vi "New Stainless Correction Pop Up 2016.vi"(3 "New Feet\n of Stainless\n(Count)":i32, 5 "Depth to \nWater Table\nInput":dbl) -> (0 "Feet of\nStainless to be\nUsed (Count)":i32, 2 "Depth to \nWater Table\nOutput":dbl)   [LabVIEW 2016]
doc: "This vi allows the clinician to input the starting flexion. It used in order to derive a flexion correction."
uses:
  KPRO_lv2015/Kpro Globals.vi
panel:
  out "Original Feet\n of Stainless\n(Count)":i32
  in  "stop":bool
  in  "Increment Stainless":bool
  in  "Stainless OK As Is":bool
  in  "Correct Stainless":bool
  # "Please Choose \nto Correct, Increment, or to \nLeave Feet of Stainless as is"
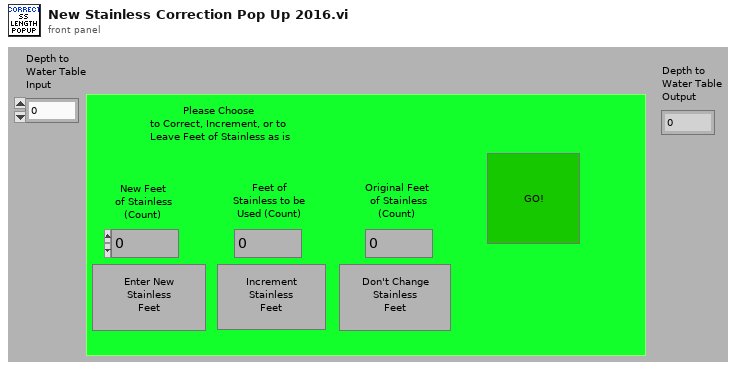
[diagram p1: front panel]
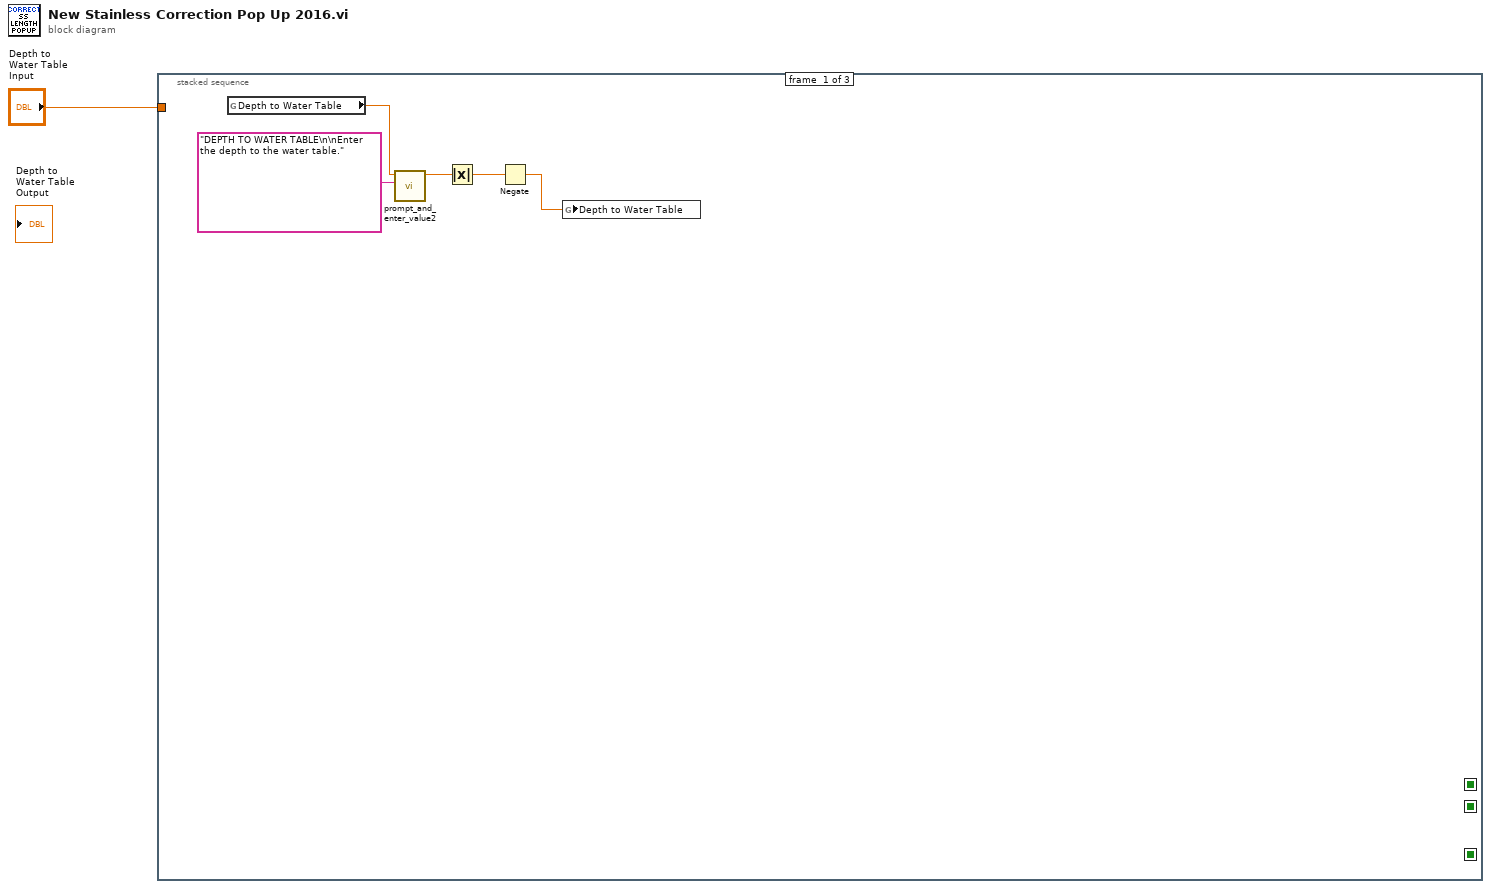
[diagram p0: block diagram]
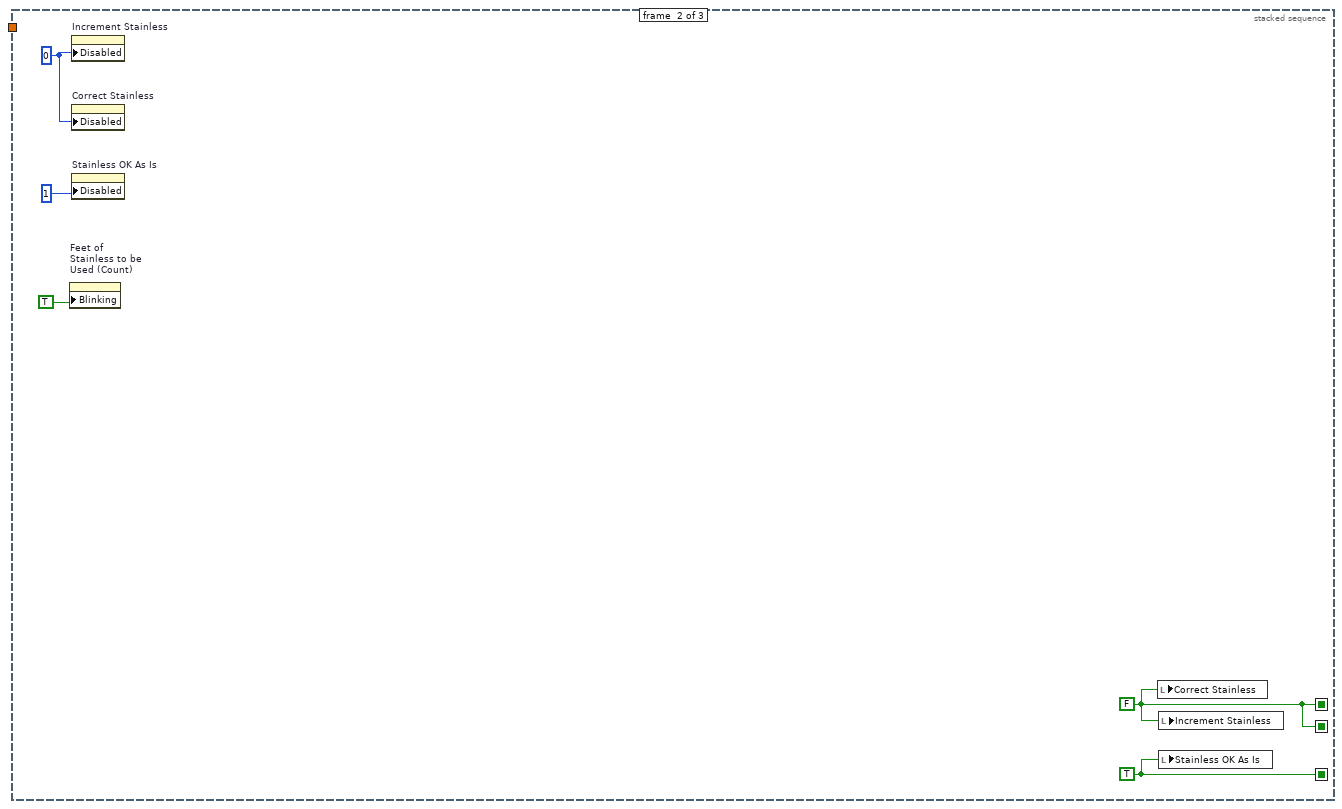
[diagram p2: hidden frame]
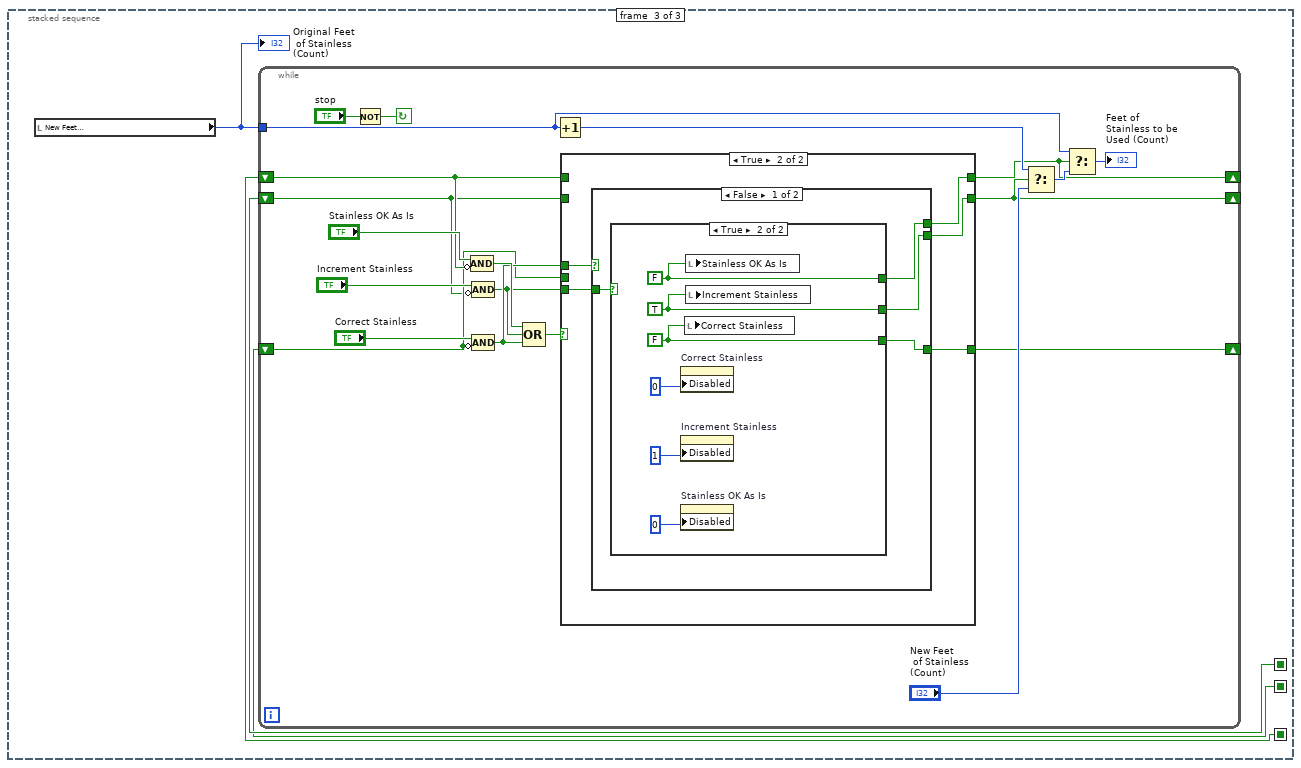
[diagram p3: hidden frame]
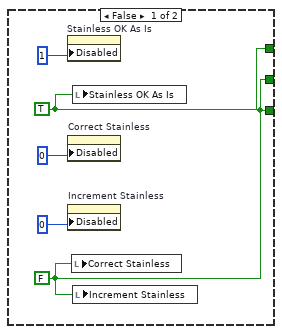
[diagram p5: hidden frame]
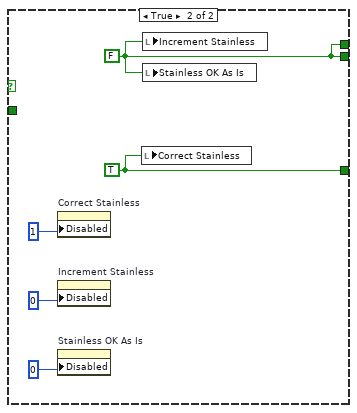
[diagram p6: hidden frame]
diagram:
  n1 = stacked-sequence {
    seq-local: [_ w10 _] -> [_ _ w13]
    seq-local: [_ w10 _] -> [_ _ w14]
    seq-local: [_ w11 _] -> [_ _ w15]
    tunnel: "Depth to \nWater Table\nInput" -> [_ _ _]
    frame #0 {
      n2 = global read "Kpro Globals.vi" "Depth to Water Table"() -> (w6:dbl)
      n3 = call "prompt_and_enter_value2.vi"("prompt_IN"="DEPTH TO WATER TABLE\n\nEnter the depth to the water table." ("prompt"), "Enter value"=w6) -> ("Numeric"=w2:dbl)  [unwired: 9 in]
      n4 = Absolute Value(x=w2) -> (abs(x)=w3:dbl)
      n5 = Negate(x=w3) -> (-x=w4:dbl)
      n6 = global write "Kpro Globals.vi" "Depth to Water Table"(w4) -> ()
    }
    frame #1 {
      w8 = 0
      w11 = TRUE
      w10 = FALSE
      n7 = property on="Feet of\nStainless to be\nUsed (Count)" class="DigNum (strict)"("Blinking"=TRUE) -> ()  [unwired: 2 in, 2 out]
      n8 = property on="Increment Stainless" class="Bool (strict)"("Disabled"=w8) -> ()  [unwired: 2 in, 2 out]
      n9 = property on="Correct Stainless" class="Bool (strict)"("Disabled"=w8) -> ()  [unwired: 2 in, 2 out]
      n10 = property on="Stainless OK As Is" class="Bool (strict)"("Disabled"=1) -> ()  [unwired: 2 in, 2 out]
      n11 = local write "Correct Stainless"(w10) -> ()
      n12 = local write "Increment Stainless"(w10) -> ()
      n13 = local write "Stainless OK As Is"(w11) -> ()
    }
    frame #2 {
      n14 = local read "New Feet\n of Stainless\n(Count)"() -> (w12:i32)
      "Original Feet\n of Stainless\n(Count)" <- w12
      n15 = while {
        tunnel: w12 -> [w17]
        shift-left: w13 -> [w19]
        shift-right: [w24] -> _
        shift-left: w14 -> [w18]
        shift-right: [w25] -> _
        shift-left: w15 -> [w20]
        shift-right: [w16] -> _
        stop <- w21 continue-if-true
        n16 = Not(x="stop") -> (.not. x?=w21:bool)
        n17 = Compound Arithmetic op=AND("Stainless OK As Is", invert w20) -> (w27:bool)
        n18 = Compound Arithmetic op=AND("Increment Stainless", invert w18) -> (w22:bool)
        n19 = Compound Arithmetic op=AND("Correct Stainless", invert w19) -> (w23:bool)
        n20 = Compound Arithmetic op=OR(w27, w22, w23) -> (w26:bool)
        n21 = Increment(x=w17) -> (x+1=w34:i32)
        n22 = case shown="True" w26 {
          tunnel: [w38 w41] -> w16
          tunnel: [w37 w40] -> w25
          tunnel: [w36 w42] -> w24
          tunnel: w23 -> [_ w43]
          tunnel: w22 -> [_ w39]
          tunnel: w20 -> [w38 _]
          tunnel: w19 -> [w36 _]
          tunnel: w18 -> [w37 _]
          frame False {
          }
          frame True {
            n23 = case shown="False" w43 {
              tunnel: [w44 w63] -> w42
              tunnel: [w46 w62] -> w41
              tunnel: [w45 w62] -> w40
              tunnel: w39 -> [w47 _]
              frame False {
                n24 = case shown="True" w47 {
                  tunnel: [w51 w56] -> w46
                  tunnel: [w52 w57] -> w45
                  tunnel: [w52 w58] -> w44
                  frame False {
                    w51 = TRUE
                    w52 = FALSE
                    n25 = property on="Stainless OK As Is" class="Bool (strict)"("Disabled"=1) -> ()  [unwired: 2 in, 2 out]
                    n26 = property on="Correct Stainless" class="Bool (strict)"("Disabled"=0) -> ()  [unwired: 2 in, 2 out]
                    n27 = property on="Increment Stainless" class="Bool (strict)"("Disabled"=0) -> ()  [unwired: 2 in, 2 out]
                    n28 = local write "Correct Stainless"(w52) -> ()
                    n29 = local write "Stainless OK As Is"(w51) -> ()
                    n30 = local write "Increment Stainless"(w52) -> ()
                  }
                  frame True {
                    w56 = FALSE
                    w57 = TRUE
                    w58 = FALSE
                    n31 = property on="Correct Stainless" class="Bool (strict)"("Disabled"=0) -> ()  [unwired: 2 in, 2 out]
                    n32 = property on="Increment Stainless" class="Bool (strict)"("Disabled"=1) -> ()  [unwired: 2 in, 2 out]
                    n33 = property on="Stainless OK As Is" class="Bool (strict)"("Disabled"=0) -> ()  [unwired: 2 in, 2 out]
                    n34 = local write "Correct Stainless"(w58) -> ()
                    n35 = local write "Stainless OK As Is"(w56) -> ()
                    n36 = local write "Increment Stainless"(w57) -> ()
                  }
                }
              }
              frame True {
                w62 = FALSE
                w63 = TRUE
                n37 = property on="Correct Stainless" class="Bool (strict)"("Disabled"=1) -> ()  [unwired: 2 in, 2 out]
                n38 = property on="Increment Stainless" class="Bool (strict)"("Disabled"=0) -> ()  [unwired: 2 in, 2 out]
                n39 = property on="Stainless OK As Is" class="Bool (strict)"("Disabled"=0) -> ()  [unwired: 2 in, 2 out]
                n40 = local write "Correct Stainless"(w63) -> ()
                n41 = local write "Increment Stainless"(w62) -> ()
                n42 = local write "Stainless OK As Is"(w62) -> ()
              }
            }
          }
        }
        n43 = Select(t=w34, s=w25, f="New Feet\n of Stainless\n(Count)") -> (s? t:f=w33:i32)
        n44 = Select(t=w17, s=w16, f=w33) -> (s? t:f=→"Feet of\nStainless to be\nUsed (Count)":i32)
      }
    }
  }
